vi "GetSetNotifierQueue.vi"(3 "Name":enum16{"topic", "node"}(ring)=enum."node", 4 "Command":string, 5 "ROS":T1={"topic port"=0, "Node"="", "topic"="", "type"="", "node port"=0, "error "={"status"=FALSE, "code"=0, "source"=""}, "Direction"=enum."Node", "APIs"=[], "Update (ms)"=1, "write queue"=1}) -> (0 "error out":errorcluster, 1 "MyState":T4, 2 "Log":T3)   [LabVIEW 2012]
uses:
  <userlib>/ROSforLV/ROS/Code/Console/Servers/ServerSubs/MyState.ctl
  <userlib>/ROSforLV/ROS/Code/Console/Servers/ServerSubs/ROSLog.ctl
  <userlib>/ROSforLV/ROS/Code/SubVIs/_ROSControl.ctl
  <userlib>/ROSforLV/ROS/Code/SubVIs/_ROSDirection.ctl
  <userlib>/ROSforLV/ROS/Code/_ROSDefinition.vi
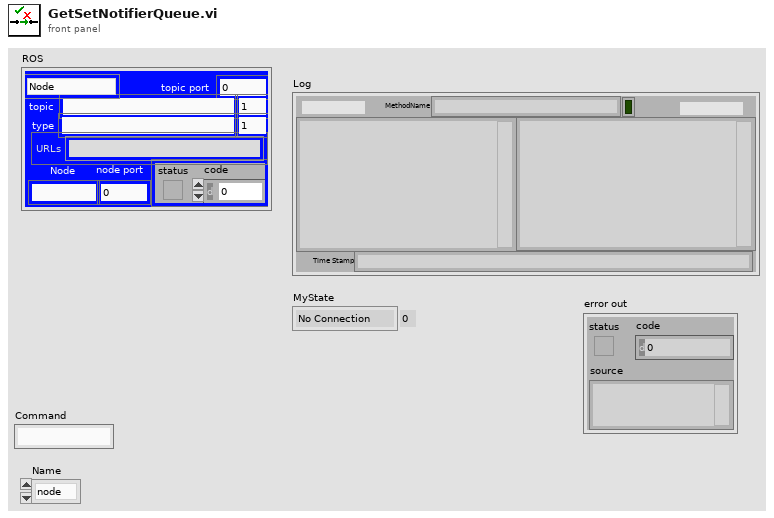
[diagram p1: front panel]
types:
  T1 = typedef "_ROSControl.ctl" = cluster{"topic port":u16, "Node":string, "topic":string, "type":string, "node port":u32, "error ":errorcluster, "Direction":T2, "APIs":string[], "Update (ms)":u16, "write queue":u16}
  T2 = typedef "_ROSDirection.ctl" = enum16{"Node", "Publisher", "Subscriber", "Service Client"}
  T3 = typedef "ROSLog.ctl" = cluster{"Sent":string, "Reply":string, "MethodName":string, "success":bool, "Dir1":string, "Dir2":string, "Time Stamp":string}
  T4 = typedef "MyState.ctl" = enum16{"No Connection", "Registered", "Connected", "Close"}
  T5 = typedef "ServoInfo.ctl" = cluster{"vi name":string, "VI Refnum":refnum<vi>, "queue":refnum<queue>, "ROS":T1, "notifier":refnum<notifier>}
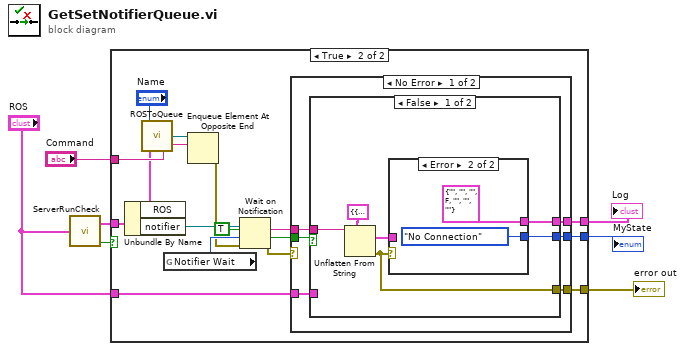
[diagram p0: block diagram]
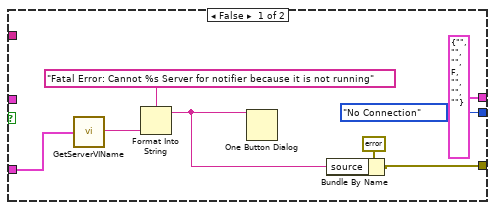
[diagram p2: hidden frame]
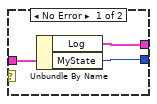
[diagram p3: hidden frame]
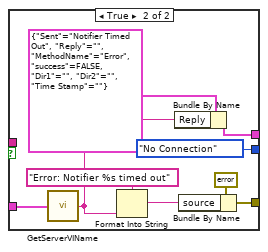
[diagram p4: hidden frame]
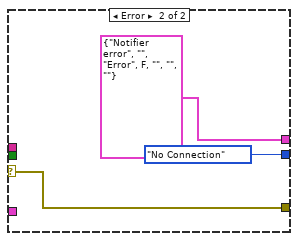
[diagram p5: hidden frame]
diagram:
  n1 = call <userlib>:"ServerRunCheck.vi"("ROS in"="ROS") -> ("Running?"=w4:bool, "ServerFound"=w3:T5)
  n2 = case shown="True" w4 {
    tunnel: w3 -> [_ w27]
    tunnel: "Command" -> [_ w22]
    tunnel: [T3 {"Sent"="", "Reply"="", "MethodName"="", "success"=FALSE, "Dir1"="", "Dir2"="", "Time Stamp"=""} ("Log") w25] -> w6
    tunnel: [MyState."No Connection" ("MyState") w24] -> w7
    tunnel: "ROS" -> [w8 w20]
    tunnel: [w9 w17] -> w2
    frame False {
      n3 = call <userlib>:"GetServerVIName.vi"("ROS"=w8) -> ("vi name"=w13:string)
      n4 = Format Into String(format string="Fatal Error: Cannot %s Server for notifier because it is not running" ("message"), w13) -> (resulting string=w10:string)  [unwired: 2 in, 1 out]
      n5 = One Button Dialog(message=w10) -> ()  [unwired: 1 in, 1 out]
      n6 = Bundle By Name(cluster=errorcluster {"status"=TRUE, "code"=0, "source"=""} ("error IO"), "source"=w10) -> (w9:errorcluster)
    }
    frame True {
      n7 = Unbundle By Name(w27) -> ("ROS"=w16:T1, "notifier"=w26:refnum<notifier>)
      n8 = call <userlib>:"ROSToQueue.vi"("ROS"=w16, "Name"="Name") -> ("queue"=w23:refnum<queue>)  [unwired: 2 in, 1 out]
      n9 = global read "_ROSDefinition.vi" "Notifier Wait"() -> (w21:i32)
      n10 = Enqueue Element At Opposite End(queue=w23, element=w22) -> (error out=w19:errorcluster)  [unwired: 2 in, 2 out]
      n11 = Wait on Notification(notifier=w26, ignore previous (F)=TRUE, timeout in ms (-1)=w21, error in (no error)=w19) -> (notification=w29:string, timed out?=w30:bool, error out=w18:errorcluster)  [unwired: 1 out]
      n12 = case shown="No Error" w18 {
        selector: w18 -> [_ w60]
        tunnel: w30 -> [w37 _]
        tunnel: w29 -> [w36 _]
        tunnel: [w35 T3 {"Sent"="Notifier error", "Reply"="", "MethodName"="Error", "success"=FALSE, "Dir1"="", "Dir2"="", "Time Stamp"=""} ("Log")] -> w25
        tunnel: [w34 MyState."No Connection" ("MyState")] -> w24
        tunnel: w20 -> [w33 _]
        tunnel: [w32 w60] -> w17
        frame No Error {
          n13 = case shown="False" w37 {
            tunnel: w36 -> [w43 _]
            tunnel: [w41 MyState."No Connection" ("MyState")] -> w34
            tunnel: [w40 w54] -> w35
            tunnel: w33 -> [_ w56]
            tunnel: [w39 w52] -> w32
            frame False {
              n14 = Unflatten From String(type=cluster{"Log":T3, "MyState":T4} {"Log"={"Sent"="", "Reply"="", "MethodName"="", "success"=FALSE, "Dir1"="", "Dir2"="", "Time Stamp"=""}, "MyState"=enum."No Connection"} ("output cluster"), binary string=w43) -> (value=w42:cluster{"Log":T3, "MyState":T4}, error out=w39:errorcluster)  [unwired: 3 in, 1 out]
              n15 = case shown="Error" w39 {
                tunnel: w42 -> [w46 _]
                tunnel: [w45 MyState."No Connection" ("MyState")] -> w41
                tunnel: [w44 T3 {"Sent"="", "Reply"="", "MethodName"="", "success"=FALSE, "Dir1"="", "Dir2"="", "Time Stamp"=""} ("Log")] -> w40
                frame No Error {
                  n16 = Unbundle By Name(w46) -> ("Log"=w44:T3, "MyState"=w45:T4)
                }
                frame Error {
                }
              }
            }
            frame True {
              n17 = call <userlib>:"GetServerVIName.vi"("ROS"=w56) -> ("vi name"=w51:string)
              n18 = Format Into String(format string="Error: Notifier %s timed out" ("MethodName"), w51) -> (resulting string=w49:string)  [unwired: 2 in, 1 out]
              n19 = Bundle By Name(cluster=T3 {"Sent"="Notifier Timed Out", "Reply"="", "MethodName"="Error", "success"=FALSE, "Dir1"="", "Dir2"="", "Time Stamp"=""} ("Log"), "Reply"=w51) -> (w54:T3)
              n20 = Bundle By Name(cluster=errorcluster {"status"=TRUE, "code"=0, "source"=""} ("error IO"), "source"=w49) -> (w52:errorcluster)
            }
          }
        }
        frame Error {
        }
      }
    }
  }
  "MyState" <- w7
  "Log" <- w6
  "error out" <- w2
